vi "Plugin FWLoader.vi"(4 "error in (no error)":errorcluster, 6 "Firmware file":path, 7 "Status reference":refnum<vi>) -> (0 "error out":errorcluster, 1 "client ptr":i32, 2 "connection ptr":i32, 3 "Connected":bool)   [LabVIEW 2010, in "lib1299.lvlib"]
doc: "This VI loads the firmware into the DSP and restarts the DSP.\n\nInputs:\nStatus reference - reference to the status indicator used to display messages and status.\nFirmware file - firmware file to be loaded (*.bin)\nerror in - error input cluster\n\nOutputs:\nConnected - boolean indicator for connection status (TRUE = connected)\nconnection ptr - connection pointer for the estyx system\nclient ptr - client pointer for the estyx system\nerror out - error output cluster"
uses:
  lib1299.lvlib
  Controls/FW State.ctl
panel:
  out "fw loader state":T1
  out "Status box":string
  out "Overall Progress":u8(slide) scale=0.0..7.0
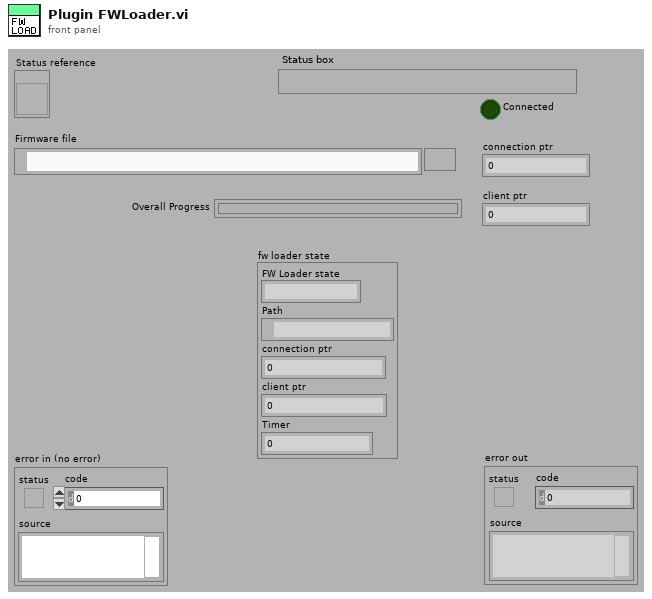
[diagram p1: front panel]
types:
  T1 = typedef "lib1299.lvlib/FW State.ctl" = cluster{"FW Loader state":string, "Path":path, "connection ptr":i32, "client ptr":i32, "Timer":i64}
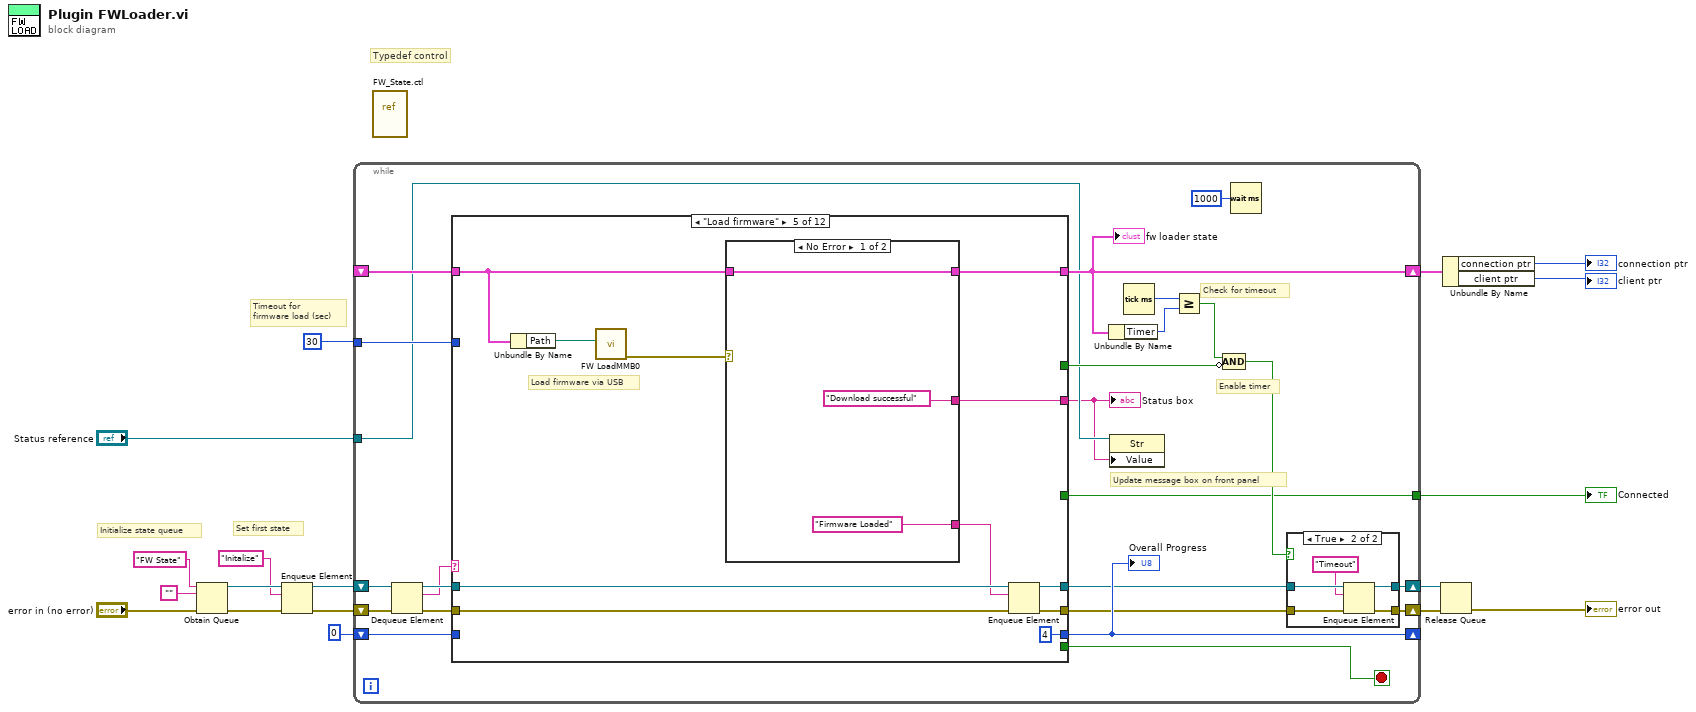
[diagram p0: block diagram]
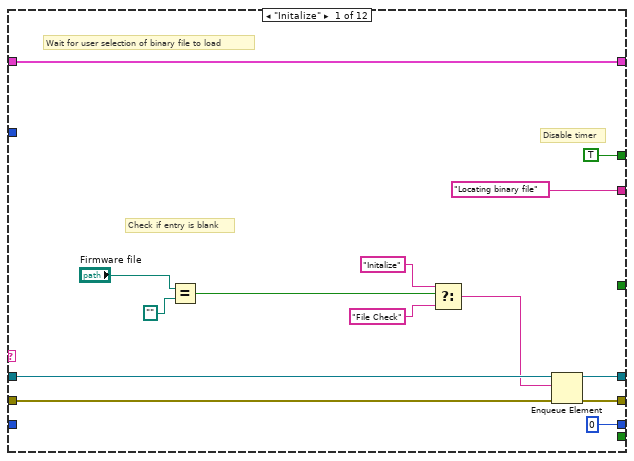
[diagram p3: hidden frame]
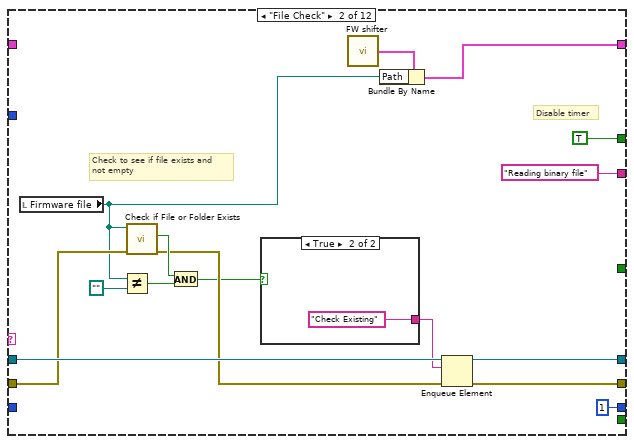
[diagram p4: hidden frame]
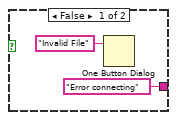
[diagram p5: hidden frame]
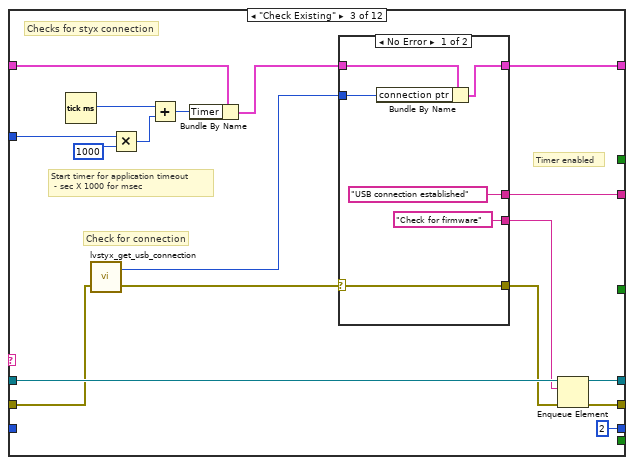
[diagram p6: hidden frame]
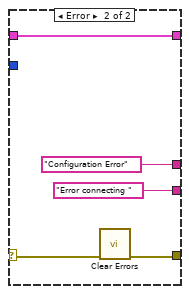
[diagram p7: hidden frame]
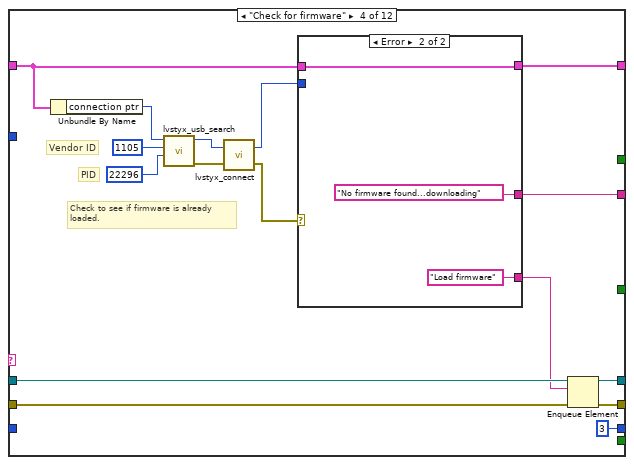
[diagram p8: hidden frame]
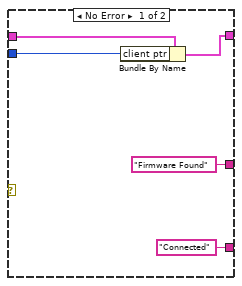
[diagram p9: hidden frame]
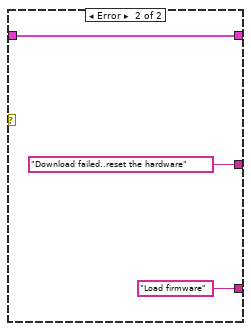
[diagram p10: hidden frame]
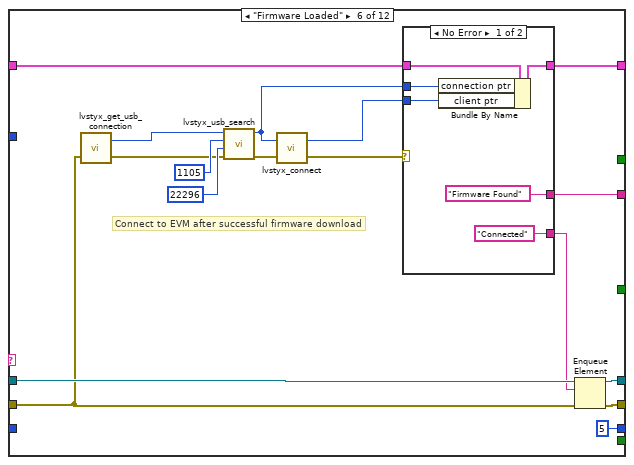
[diagram p11: hidden frame]
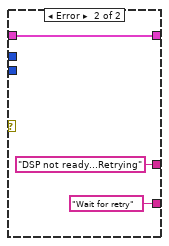
[diagram p12: hidden frame]
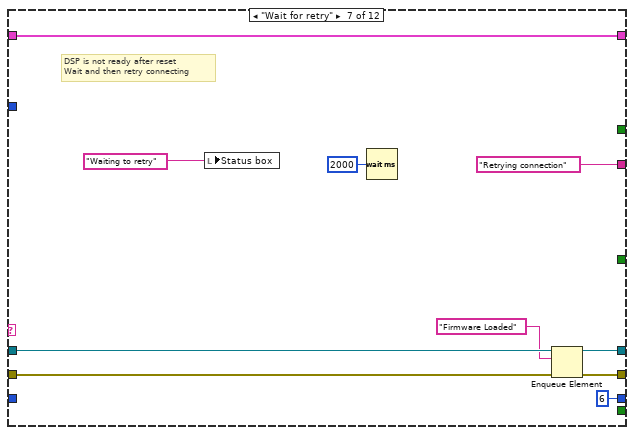
[diagram p13: hidden frame]
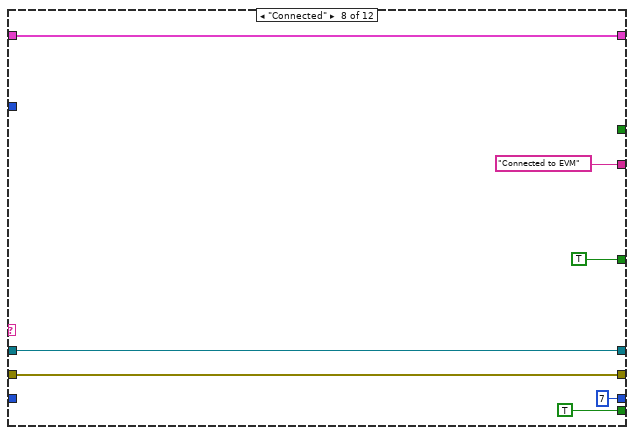
[diagram p14: hidden frame]
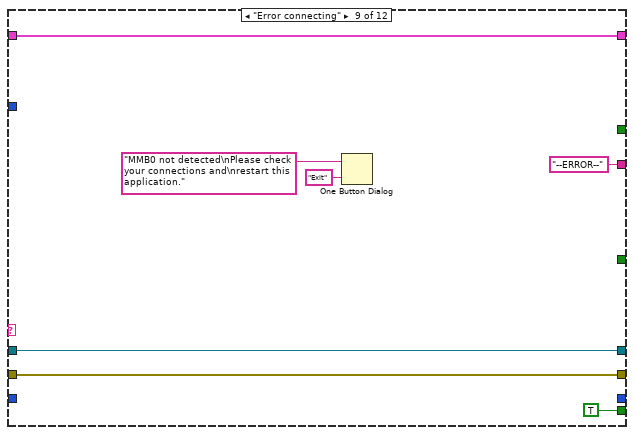
[diagram p15: hidden frame]
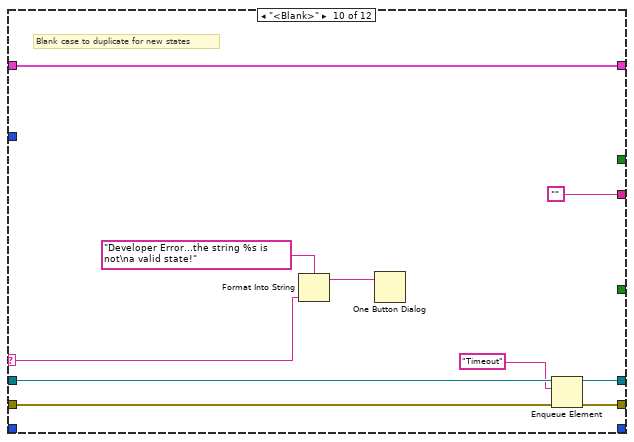
[diagram p16: hidden frame]
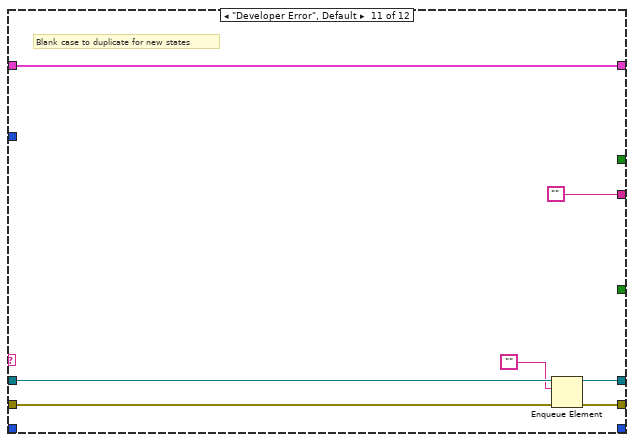
[diagram p17: hidden frame]
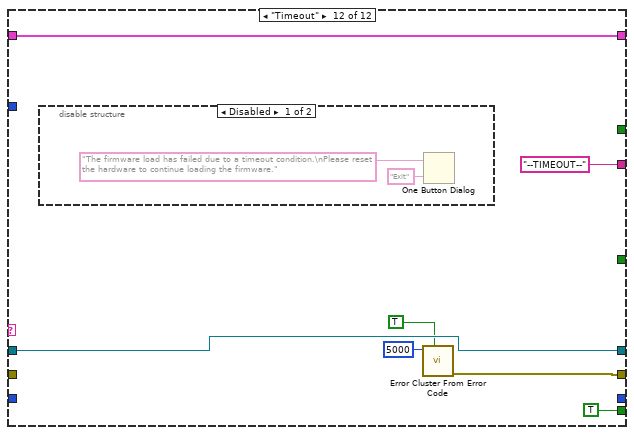
[diagram p18: hidden frame]
diagram:
  # "Typedef control"
  # "Set first state"
  # "Initialize state queue"
  # "Timeout for\nfirmware load (sec)"
  n1 = Obtain Queue(name (unnamed)="FW State", element data type="", error in (no error)="error in (no error)") -> (queue out=w18:refnum<queue>, error out=w17:errorcluster)  [unwired: 2 in, 1 out]
  n2 = Enqueue Element(queue=w18, element="Initalize", error in (no error)=w17) -> (queue out=w16:refnum<queue>, error out=w12:errorcluster)  [unwired: 1 in, 1 out]
  n3 = while {
    shift-right: [w35] -> w6
    shift-left: _ -> [w36]
    shift-right: [w23] -> w11
    shift-left: w12 -> [w37]
    shift-right: [w24] -> w10
    shift-left: w16 -> [w42]
    tunnel: 30 ("y") -> [w34]
    shift-right: [w28] -> _
    shift-left: 0 -> [w29]
    tunnel: "Status reference" -> [w21]
    tunnel: [w19] -> w1
    stop <- w27 stop-if-true
    # "Update message box on front panel"
    # "Enable timer"
    # "Check for timeout"
    n4 = Dequeue Element(queue=w42, error in (no error)=w37) -> (queue out=w41:refnum<queue>, element=w40:string, error out=w39:errorcluster)  [unwired: 1 in, 1 out]
    n5 = case shown="\"Load firmware\"" w40 {
      selector: w40 -> [_ _ _ _ _ _ _ _ _ w204 _ _]
      tunnel: w41 -> [w61 w76 w98 w125 w144 w167 w186 w195 w199 w210 w217 w225]
      tunnel: w39 -> [w60 w72 w97 w124 w143 w162 w185 w194 w198 w209 w216 _]
      tunnel: [w63 w75 w100 w127 w146 w169 w188 w195 w199 w212 w219 w225] -> w26
      tunnel: [w59 w73 w93 w114 w138 w156 w184 w191 w202 w207 w213 w226] -> w35
      tunnel: [w62 w68 w99 w126 w145 w168 w187 w194 w198 w211 w218 w222] -> w25
      tunnel: w36 -> [w59 _ w86 w115 w137 w157 w184 w191 w202 w207 w213 w226]
      tunnel: ["Locating binary file" "Reading binary file" w91 w116 w140 w155 "Retrying connection" "Connected to EVM" "--ERROR--" "" "" "--TIMEOUT--"] -> w20
      tunnel: [_ _ _ _ _ _ _ TRUE TRUE _ _ TRUE] -> w27
      tunnel: w34 -> [_ _ w87 _ _ _ _ _ _ _ _ _]
      tunnel: [TRUE TRUE _ _ _ _ _ _ _ _ _ _] -> w31
      tunnel: w29 -> [_ _ _ _ _ _ _ _ _ _ _ _]
      tunnel: [0 1 2 3 4 5 6 7 _ _ _ _] -> w28
      tunnel: [_ _ _ _ _ _ _ TRUE _ _ _ _] -> w19
      frame "Initalize" {
        # "Disable timer"
        # "Check if entry is blank"
        # "Wait for user selection of binary file to load"
        n6 = Equal?(x="Firmware file", y=path "") -> (x = y?=w53:bool)
        n7 = Select(t="Initalize", s=w53, f="File Check") -> (s? t:f=w55:string)
        n8 = Enqueue Element(queue=w61, element=w55, error in (no error)=w60) -> (queue out=w63:refnum<queue>, error out=w62:errorcluster)  [unwired: 1 in, 1 out]
      }
      frame "File Check" {
        # "Check to see if file exists and\nnot empty"
        # "Disable timer"
        n9 = local read "Firmware file"() -> (w65:path)
        n10 = Not Equal?(x=w65, y=path "") -> (x != y?=w79:bool)
        n11 = call <vilib>:"Check if File or Folder Exists.vi"("error in (no error)"=w72, "path"=w65) -> ("error out"=w71:errorcluster, "file or folder exists?"=w78:bool)  [unwired: 7 in, 1 out]
        n12 = And(x=w78, y=w79) -> (x .and. y?=w70:bool)
        n13 = case shown="True" w70 {
          tunnel: ["Error connecting" "Check Existing"] -> w69
          frame False {
            n14 = One Button Dialog(message="Invalid File") -> ()  [unwired: 1 in, 1 out]
          }
          frame True {
          }
        }
        n15 = call "FW shifter.vi"() -> ("Cluster"=w74:T1)  [unwired: 1 in]
        n16 = Bundle By Name(cluster=w74, "Path"=w65) -> (w73:T1)
        n17 = Enqueue Element(queue=w76, element=w69, error in (no error)=w71) -> (queue out=w75:refnum<queue>, error out=w68:errorcluster)  [unwired: 1 in, 1 out]
      }
      frame "Check Existing" {
        # "Timer enabled"
        # "Checks for styx connection"
        # "Check for connection"
        # "Start timer for application timeout\n - sec X 1000 for msec"
        n18 = Tick Count (ms)() -> (millisecond timer value=w89:u32)
        n19 = call "lvstyx_get_usb_connection.vi"("error in (no error)"=w97) -> ("error out"=w96:errorcluster, "connection ptr"=w92:u32)  [unwired: 1 in]
        n20 = Multiply(x=w87, y=1000) -> (x*y=w90:i32)
        n21 = Add(x=w89, y=w90) -> (x+y=w84:u32)
        n22 = Bundle By Name(cluster=w86, "Timer"=w84) -> (w85:T1)
        n23 = case shown="No Error" w96 {
          selector: w96 -> [w106 w110]
          tunnel: [w106 w111] -> w95
          tunnel: ["Check for firmware" "Error connecting "] -> w94
          tunnel: w85 -> [w102 w107]
          tunnel: [w101 w107] -> w93
          tunnel: w92 -> [w103 _]
          tunnel: ["USB connection established" "Configuration Error"] -> w91
          frame No Error {
            n24 = Bundle By Name(cluster=w102, "connection ptr"=w103) -> (w101:T1)
          }
          frame Error {
            n25 = call <vilib>:"Clear Errors.vi"("error in (no error)"=w110) -> ("error out"=w111:errorcluster)  [unwired: 6 in]
          }
        }
        n26 = Enqueue Element(queue=w98, element=w94, error in (no error)=w95) -> (queue out=w100:refnum<queue>, error out=w99:errorcluster)  [unwired: 1 in, 1 out]
      }
      frame "Check for firmware" {
        # "PID"
        # "Vendor ID"
        # "Check to see if firmware is already\nloaded."
        n27 = Unbundle By Name(w115) -> ("connection ptr"=w120:i32)
        n28 = call "lvstyx_usb_search.vi"("pid"=u16 22296, "vid"=u16 1105, "conn ptr"=w120) -> ("error out"=w122:errorcluster, "dup conn ptr"=w118:u32)  [unwired: 6 in, 1 out]
        n29 = call "lvstyx_connect.vi"("error in (no error)"=w122, "connection ptr"=w118) -> ("error out"=w119:errorcluster, "client ptr"=w113:u32)
        n30 = case shown="Error" w119 {
          tunnel: ["Connected" "Load firmware"] -> w117
          tunnel: ["Firmware Found" "No firmware found...downloading"] -> w116
          tunnel: w115 -> [w130 w133]
          tunnel: [w129 w133] -> w114
          tunnel: w113 -> [w128 _]
          frame No Error {
            n31 = Bundle By Name(cluster=w130, "client ptr"=w128) -> (w129:T1)
          }
          frame Error {
          }
        }
        n32 = Enqueue Element(queue=w125, element=w117, error in (no error)=w124) -> (queue out=w127:refnum<queue>, error out=w126:errorcluster)  [unwired: 1 in, 1 out]
      }
      frame "Load firmware" {
        # "Load firmware via USB"
        n33 = Unbundle By Name(w137) -> ("Path"=w142:path)
        n34 = call "FW LoadMMB0.vi"("Boot file"=w142) -> ("error out"=w141:errorcluster)  [unwired: 10 in]
        n35 = case shown="No Error" w141 {
          tunnel: ["Download successful" "Download failed..reset the hardware"] -> w140
          tunnel: ["Firmware Loaded" "Load firmware"] -> w139
          tunnel: [w147 w152] -> w138
          tunnel: w137 -> [w147 w152]
          frame No Error {
          }
          frame Error {
          }
        }
        n36 = Enqueue Element(queue=w144, element=w139, error in (no error)=w143) -> (queue out=w146:refnum<queue>, error out=w145:errorcluster)  [unwired: 1 in, 1 out]
      }
      frame "Firmware Loaded" {
        # "Connect to EVM after successful firmware download"
        n37 = call "lvstyx_get_usb_connection.vi"("error in (no error)"=w162) -> ("error out"=w161:errorcluster, "connection ptr"=w163:u32)  [unwired: 1 in]
        n38 = call "lvstyx_usb_search.vi"("error in (no error)"=w161, "pid"=u16 22296, "vid"=u16 1105, "conn ptr"=w163) -> ("error out"=w164:errorcluster, "dup conn ptr"=w158:u32)  [unwired: 5 in, 1 out]
        n39 = call "lvstyx_connect.vi"("error in (no error)"=w164, "connection ptr"=w158) -> ("error out"=w160:errorcluster, "client ptr"=w159:u32)
        n40 = case shown="No Error" w160 {
          tunnel: w159 -> [w172 _]
          tunnel: w158 -> [w173 _]
          tunnel: w157 -> [w175 w178]
          tunnel: [w174 w178] -> w156
          tunnel: ["Firmware Found" "DSP not ready...Retrying"] -> w155
          tunnel: ["Connected" "Wait for retry"] -> w154
          frame No Error {
            n41 = Bundle By Name(cluster=w175, "connection ptr"=w173, "client ptr"=w172) -> (w174:T1)
          }
          frame Error {
          }
        }
        n42 = Enqueue Element(queue=w167, element=w154, error in (no error)=w162) -> (queue out=w169:refnum<queue>, error out=w168:errorcluster)  [unwired: 1 in, 1 out]
      }
      frame "Wait for retry" {
        # "DSP is not ready after reset\nWait and then retry connecting"
        n43 = local write "Status box"("Waiting to retry") -> ()
        n44 = Wait (ms)(milliseconds to wait=u32 2000) -> ()  [unwired: 1 out]
        n45 = Enqueue Element(queue=w186, element="Firmware Loaded", error in (no error)=w185) -> (queue out=w188:refnum<queue>, error out=w187:errorcluster)  [unwired: 1 in, 1 out]
      }
      frame "Connected" {
      }
      frame "Error connecting" {
        n46 = One Button Dialog(message="MMB0 not detected\nPlease check your connections and\nrestart this application.", button name ("OK")="Exit") -> ()  [unwired: 1 out]
      }
      frame "<Blank>" {
        # "Blank case to duplicate for new states"
        n47 = Format Into String(format string="Developer Error...the string %s is not\na valid state!", w204) -> (resulting string=w205:string)  [unwired: 2 in, 1 out]
        n48 = One Button Dialog(message=w205) -> ()  [unwired: 1 in, 1 out]
        n49 = Enqueue Element(queue=w210, element="Timeout", error in (no error)=w209) -> (queue out=w212:refnum<queue>, error out=w211:errorcluster)  [unwired: 1 in, 1 out]
      }
      frame "Developer Error", Default {
        # "Blank case to duplicate for new states"
        n50 = Enqueue Element(queue=w217, element="", error in (no error)=w216) -> (queue out=w219:refnum<queue>, error out=w218:errorcluster)  [unwired: 1 in, 1 out]
      }
      frame "Timeout" {
        n51 = disable-structure shown="Disabled" {
          frame Disabled {
            n52 = One Button Dialog(message="The firmware load has failed due to a timeout condition.\nPlease reset the hardware to continue loading the firmware.", button name ("OK")="Exit") -> ()  [unwired: 1 out]
          }
          frame Enabled {
          }
        }
        n53 = call <vilib>:"Error Cluster From Error Code.vi"("show call chain? (False)"=TRUE, "error code (0)"=5000) -> ("error out"=w222:errorcluster)  [unwired: 7 in]
      }
    }
    "fw loader state" <- w35
    "Status box" <- w20
    "Overall Progress" <- w28
    n54 = Unbundle By Name(w35) -> ("Timer"=w32:i64)
    n55 = property class="Str"(reference=w21, "Value"=w20) -> ()  [unwired: 1 in, 2 out]
    n56 = Tick Count (ms)() -> (millisecond timer value=w33:u32)
    n57 = Greater Or Equal?(x=w33, y=w32) -> (x >= y?=w30:bool)
    n58 = Compound Arithmetic op=AND(w30, invert w31) -> (w22:bool)
    n59 = Wait (ms)(milliseconds to wait=u32 1000) -> ()  [unwired: 1 out]
    n60 = case shown="True" w22 {
      tunnel: w26 -> [w44 w49]
      tunnel: w25 -> [w43 w48]
      tunnel: [w44 w47] -> w24
      tunnel: [w43 w46] -> w23
      frame False {
      }
      frame True {
        n61 = Enqueue Element(queue=w49, element="Timeout", error in (no error)=w48) -> (queue out=w47:refnum<queue>, error out=w46:errorcluster)  [unwired: 1 in, 1 out]
      }
    }
  }
  "Connected" <- w1
  n62 = vi-ref "FW_State.ctl"() -> ()  [unwired: 1 out]
  n63 = Release Queue(queue=w10, error in (no error)=w11) -> (error out=→"error out":errorcluster)  [unwired: 1 in, 2 out]
  n64 = Unbundle By Name(w6) -> ("connection ptr"=→"connection ptr":i32, "client ptr"=→"client ptr":i32)
